vi "Self-Test.vi"(8 "error in (no error)":errorcluster, 10 "Self-Test Mode (0: Run)":i32(ring) items=["Run", "Read-Only", "Clear Results"], 11 "VISA resource name":refnum<visa-resource-name>) -> (0 "error out":errorcluster, 1 "Self-Test Result Message":string, 2 "Self-Test Result Code":i32, 3 "VISA resource name out":refnum<visa-resource-name>)   [LabVIEW 2018, in "XP Power PLS600.lvlib"]
doc: "Runs the instrument's self-test routine and returns the test results. If a self-test error has occurred, the instrument must be power cycled to recover from the error condition. Also provides the option to read the results from the last self-test that was executed, or clear the self-test results."
uses:
  XP Power PLS600.lvlib
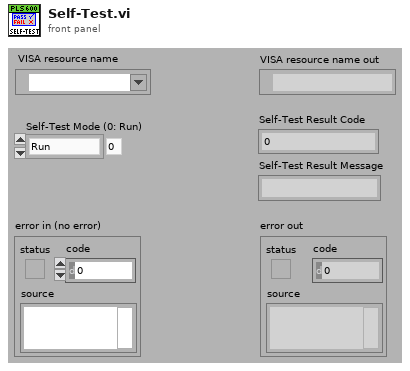
[diagram p1: front panel]
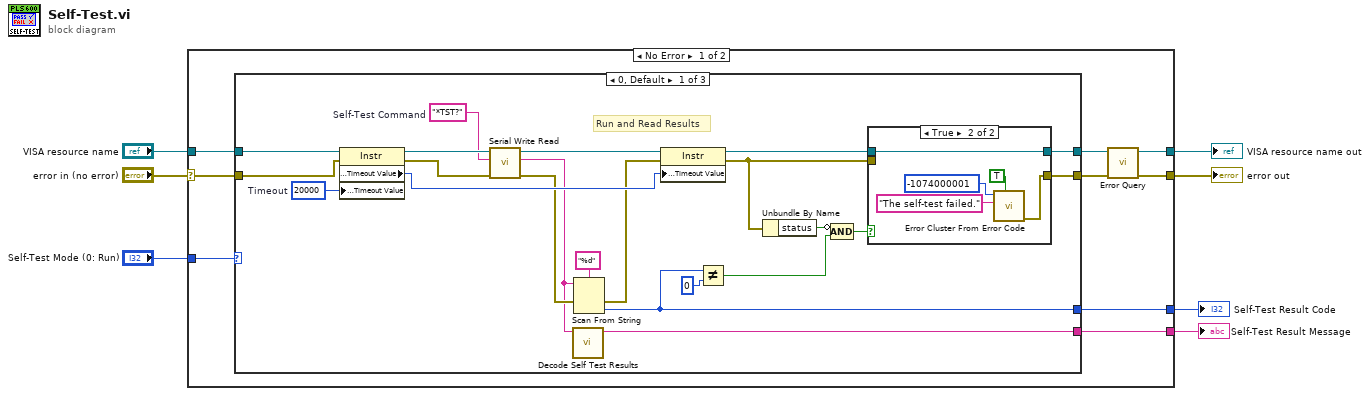
[diagram p0: block diagram]
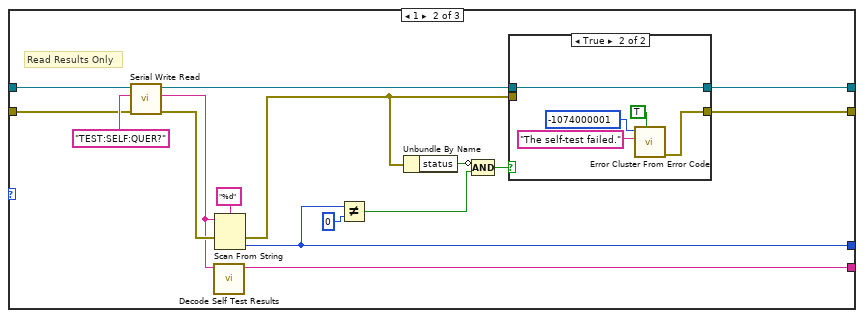
[diagram p3: hidden frame]
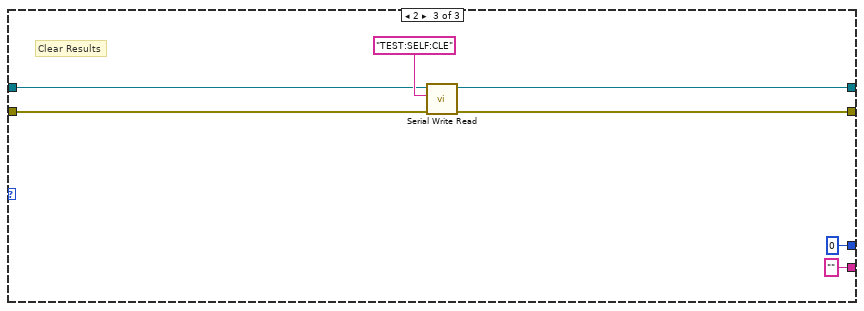
[diagram p5: hidden frame]
diagram:
  n1 = case shown="No Error" "error in (no error)" {
    selector: "error in (no error)" -> [w11 w76]
    tunnel: "VISA resource name" -> [w16 w77]
    tunnel: [w15 w77] -> w6
    tunnel: [w14 w76] -> w5
    tunnel: "Self-Test Mode (0: Run)" -> [w10 _]
    tunnel: [w9 _] -> w2
    tunnel: [w8 _] -> w1
    frame No Error {
      n2 = case shown="0, Default" w10 {
        tunnel: w16 -> [w37 w51 w73]
        tunnel: [w32 w48 w71] -> w13
        tunnel: [w31 w49 w72] -> w12
        tunnel: w11 -> [w19 w50 w74]
        tunnel: [w18 w47 0] -> w9
        tunnel: [w17 w46 "" ("Self-Test Result Message")] -> w8
        frame 0, Default {
          w36 = u32 20000  # Timeout
          w20 = "*TST?"  # Self-Test Command
          # "Run and Read Results"
          n3 = property class="Instr"(reference=w37, error in=w19, "General Settings:Timeout Value"=w36) -> (reference out=w21:refnum<visa-resource-name>, error out=w25:errorcluster, "General Settings:Timeout Value"=w35:u32)
          n4 = call "Serial Write Read.vi"("error in (no error)"=w25, "Write Buffer"=w20, "VISA resource name"=w21) -> ("error out"=w24:errorcluster, "Read Buffer"=w23:string, "VISA resource name out"=w22:refnum<visa-resource-name>)  [unwired: 6 in]
          n5 = call "Decode Self Test Results.vi"("Status"=w23) -> ("Self-Test Result Message"=w17:string)  [unwired: 10 in]
          n6 = Scan From String(format string="%d", input string=w23, error in=w24) -> (error out=w26:errorcluster, output 1=w18:i32)  [unwired: 2 in, 2 out]
          n7 = property class="Instr"(reference=w22, error in=w26, "General Settings:Timeout Value"=w35) -> (reference out=w34:refnum<visa-resource-name>, error out=w33:errorcluster)
          n8 = Not Equal?(x=w18, y=0) -> (x != y?=w30:bool)
          n9 = Unbundle By Name(w33) -> ("status"=w29:bool)
          n10 = Compound Arithmetic op=AND(invert w29, w30) -> (w28:bool)
          n11 = case shown="True" w28 {
            tunnel: w34 -> [w40 w45]
            tunnel: w33 -> [w39 _]
            tunnel: [w39 w41] -> w32
            tunnel: [w40 w45] -> w31
            frame False {
            }
            frame True {
              n12 = call <vilib>:"Error Cluster From Error Code.vi"("show call chain? (False)"=TRUE, "error message (\"\")"="The self-test failed." ("Source (VI Name)"), "error code (0)"=-1074000001 ("Code")) -> ("error out"=w41:errorcluster)  [unwired: 6 in]
            }
          }
        }
        frame 1 {
          # "Read Results Only"
          n13 = call "Serial Write Read.vi"("error in (no error)"=w50, "Write Buffer"="TEST:SELF:QUER?", "VISA resource name"=w51) -> ("error out"=w56:errorcluster, "Read Buffer"=w55:string, "VISA resource name out"=w53:refnum<visa-resource-name>)  [unwired: 6 in]
          n14 = call "Decode Self Test Results.vi"("Status"=w55) -> ("Self-Test Result Message"=w46:string)  [unwired: 10 in]
          n15 = Scan From String(format string="%d", input string=w55, error in=w56) -> (error out=w52:errorcluster, output 1=w47:i32)  [unwired: 2 in, 2 out]
          n16 = Not Equal?(x=w47, y=0) -> (x != y?=w60:bool)
          n17 = Unbundle By Name(w52) -> ("status"=w59:bool)
          n18 = Compound Arithmetic op=AND(invert w59, w60) -> (w58:bool)
          n19 = case shown="True" w58 {
            tunnel: w53 -> [w63 w68]
            tunnel: w52 -> [w62 _]
            tunnel: [w62 w64] -> w48
            tunnel: [w63 w68] -> w49
            frame False {
            }
            frame True {
              n20 = call <vilib>:"Error Cluster From Error Code.vi"("show call chain? (False)"=TRUE, "error message (\"\")"="The self-test failed." ("Source (VI Name)"), "error code (0)"=-1074000001 ("Code")) -> ("error out"=w64:errorcluster)  [unwired: 6 in]
            }
          }
        }
        frame 2 {
          # "Clear Results"
          n21 = call "Serial Write Read.vi"("error in (no error)"=w74, "Write Buffer"="TEST:SELF:CLE" ("Command to Send (empty)"), "VISA resource name"=w73) -> ("error out"=w71:errorcluster, "VISA resource name out"=w72:refnum<visa-resource-name>)  [unwired: 6 in, 1 out]
        }
      }
      n22 = call "Error Query.vi"("error in (no error)"=w13, "VISA resource name"=w12) -> ("error out"=w14:errorcluster, "VISA resource name out"=w15:refnum<visa-resource-name>)  [unwired: 6 in, 2 out]
    }
    frame Error {
    }
  }
  "VISA resource name out" <- w6
  "error out" <- w5
  "Self-Test Result Message" <- w1
  "Self-Test Result Code" <- w2
